vi "Host - extract control Ref.vi"(9 "Co-Pilot Tab":string[](array[string]), 10 "Pilot Tab":string[](array[string]), 11 "Pages":refnum<vi>[](array[refnum])) -> (1 "All Controls":refnum<vi>[](array[refnum]), 2 "Co-Pilot Controls":refnum<vi>[](array[refnum]), 3 "Pilot Controls":refnum<vi>[](array[refnum]), 4 "Propulsion:Controls":refnum<vi>[](array[refnum]))   [LabVIEW 2022 SP3]
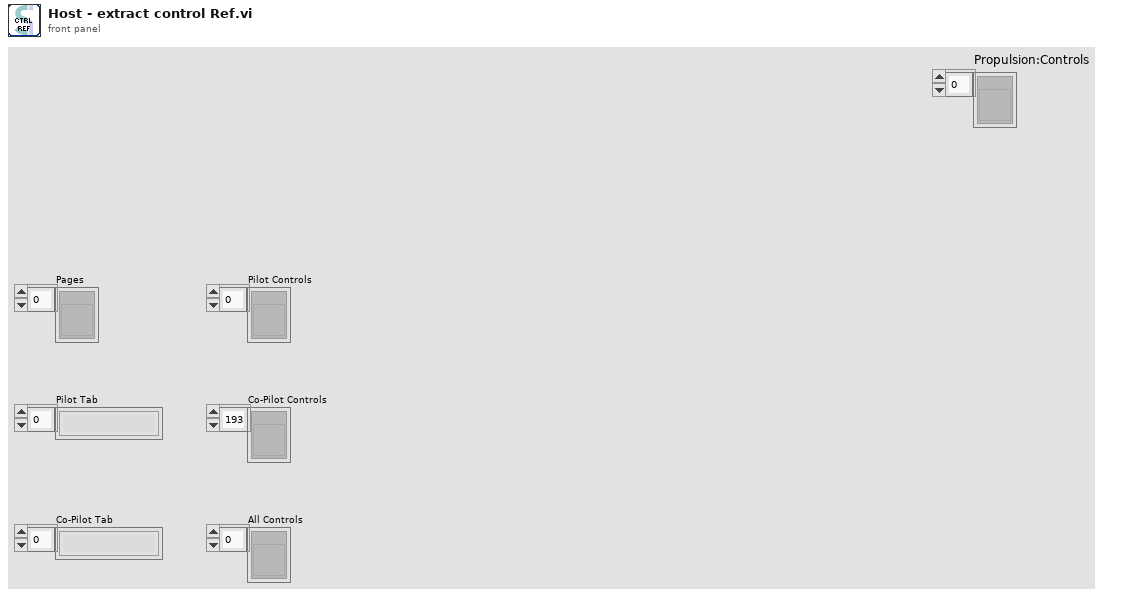
[diagram p1: front panel]
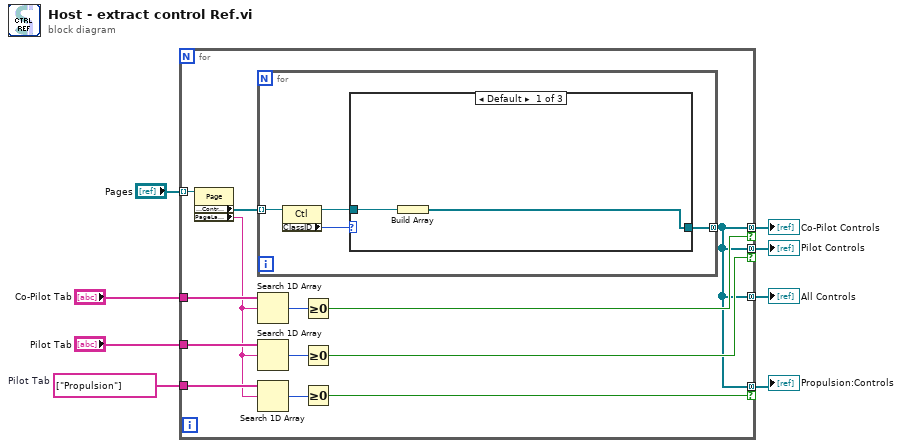
[diagram p0: block diagram]
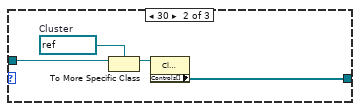
[diagram p2: hidden frame]
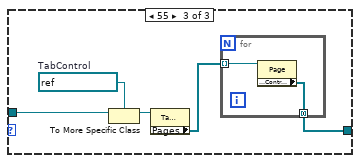
[diagram p3: hidden frame]
diagram:
  w2 = string[] ["Propulsion"]  # Pilot Tab
  n1 = for {
    tunnel: "Pages" -> [w14] mode=indexing
    tunnel: [w11] -> w4 mode=concatenating if=w15
    tunnel: "Pilot Tab" -> [w21]
    tunnel: "Co-Pilot Tab" -> [w20]
    tunnel: [w11] -> w3 mode=concatenating if=w17
    tunnel: [w11] -> w8 mode=concatenating
    tunnel: w2 -> [w13]
    tunnel: [w11] -> w1 mode=concatenating if=w10
    n2 = property class="Page"(reference=w14) -> ("Z-Order:Controls[]"=w16:refnum<vi>[], "PageLabel"=w9:string)  [unwired: 1 in, 2 out]
    n3 = for {
      tunnel: w16 -> [w25] mode=indexing
      tunnel: [w22] -> w11 mode=concatenating
      n4 = property on="Property Node" class="Ctl"(reference=w25) -> (reference out=w23:refnum<vi>, "ClassID"=w24:u32)  [unwired: 1 in, 1 out]
      n5 = case shown="Default" w24 {
        tunnel: w23 -> [w27 w31 w36]
        tunnel: [w26 w28 w32] -> w22
        frame Default {
          n6 = Build Array(w27) -> (w26:refnum<vi>[])
        }
        frame 30 {
          w29 = refnum<vi> refnum  # Cluster
          n7 = To More Specific Class(target class=w29, reference=w31) -> (specific class reference=w30:refnum<vi>)  [unwired: 1 in, 1 out]
          n8 = property class="Clust"(reference=w30) -> ("Controls[]"=w28:refnum<vi>[])  [unwired: 1 in, 2 out]
        }
        frame 55 {
          w34 = refnum<vi> refnum  # TabControl
          n9 = To More Specific Class(target class=w34, reference=w36) -> (specific class reference=w35:refnum<vi>)  [unwired: 1 in, 1 out]
          n10 = property class="TabCtl"(reference=w35) -> ("Pages"=w33:refnum<vi>[])  [unwired: 1 in, 2 out]
          n11 = for {
            tunnel: w33 -> [w38] mode=indexing
            tunnel: [w37] -> w32 mode=concatenating
            n12 = property class="Page"(reference=w38) -> ("Z-Order:Controls[]"=w37:refnum<vi>[])  [unwired: 1 in, 2 out]
          }
        }
      }
    }
    n13 = Search 1D Array(1D array=w20, element=w9) -> (index of element=w18:i32)  [unwired: 1 in]
    n14 = Search 1D Array(1D array=w21, element=w9) -> (index of element=w19:i32)  [unwired: 1 in]
    n15 = Search 1D Array(1D array=w13, element=w9) -> (index of element=w12:i32)  [unwired: 1 in]
    n16 = Greater Or Equal To 0?(x=w18) -> (x >= 0?=w17:bool)
    n17 = Greater Or Equal To 0?(x=w19) -> (x >= 0?=w15:bool)
    n18 = Greater Or Equal To 0?(x=w12) -> (x >= 0?=w10:bool)
  }
  "All Controls" <- w8
  "Co-Pilot Controls" <- w3
  "Pilot Controls" <- w4
  "Propulsion:Controls" <- w1
